vi "Demo_Main0.vi"() -> ()   [LabVIEW 2010]
uses:
  ControlCAN/ControlCAN.llb/DevType.ctl
  ControlCAN/ControlCAN.llb/CAN Channel.ctl
  ControlCAN/ControlCAN.llb/InitFlag.ctl
  ControlCAN/ControlCAN.llb/Mode.ctl
  ControlCAN/ControlCAN.llb/Fliter.ctl
  ControlCAN/ControlCAN.llb/VCI_CAN_OBJ.ctl
  ControlCAN/ControlCAN.llb/VCI_INIT_CONFIG.ctl
  ControlCAN/ControlCAN.llb/Return Val.ctl
  ControlCAN/ControlCAN.lvlib
panel:
  out "sCnt":u32 caption="处理统计"
  out "模式_回":string(combo)="00"
  in  "模式_R":bool
  in  "设定电流_R":bool
  in  "设定位置_R":bool
  in  "设定速度_R":bool
  in  "存储路径":path
  in  "保存":bool
  out "保存_S":bool
  in  "模式_W":bool
  in  "模式":string(combo)="00"
  in  "设定电流":dbl format="%#.6f"
  out "设定电流_回":dbl format="%#.6f"
  in  "设定电流_W":bool
  in  "设定位置":dbl format="%#.6f"
  out "设定位置_回":dbl format="%#.6f"
  in  "设定位置_W":bool
  in  "设定速度":dbl format="%#.1f"
  out "设定速度_回":dbl format="%#.6f"
  in  "设定速度_W":bool
  in  "监测_W":bool
  in  "监测":string(combo)="30"
  out "电机ID_R":u32
  in  "Clear":bool
  out "Ualfa":dbl format="%#.6f"
  out "Ubate":dbl format="%#.6f"
  out "Uq":dbl format="%#.6f"
  out "Ud":dbl format="%#.6f"
  out "PWM1":u16
  out "PWM2":u16
  out "PWM3":u16
  out "sector":u8
  out "Iqnow":dbl
  out "Idnow":dbl
  out "Ialfa":dbl
  out "Ibeta":dbl
  out "A电流":dbl
  out "C电流":dbl
  out "B电流":dbl
  out "供电电压":dbl
  out "机械角度":dbl format="%.2f"
  out "电气角度":dbl
  out "转速":dbl
  out "CAN STD_ID":u32 format="%x"
  in  "电机ID":string(combo)="00"
  in  "电机ID_W":bool
  out "RecvCnt":u32 caption="接收统计"
  out "SendCnt":u32 caption="发送统计"
  in  "Format":u8(ring) items=["标准帧", "扩展帧"]
  in  "Type":u8(ring) items=["数据帧", "远程帧"]
  in  "Data":string="00 01 02 03 04 05 06 07"
  in  "ID":u32=291 format="0x%x"
  in  "Send":bool
  in  "RcvEnable":bool=TRUE
  out "Open":bool
  in  "Fliter":T1=1 items=["接收所有类型"=1, "只接收标准帧"=2, "只接收扩展帧"=3]
  in  "kBaudRate":u8(ring)=12 caption="波特率" items=["5k bps"=1, "10k bps"=2, "20k bps"=3, "40k bps"=4, "50k bps"=5, "80k bps"=6, "100k bps"=7, "125k bps"=8, "200k bps"=9, "250k bps"=10, "400k bps"=11, "500k bps"=12, "666k bps"=13, "800k bps"=14, "1000k bps"=15, "33.33k bps"=16, "66.66k bps"=17, "83.33k bps"=18]
  in  "Mode":T2 caption="工作模式" items=["正常工作", "仅侦听模式", "自测模式（环回）"]
  in  "InitFlag":T3 caption="初始化参数" items=["使用Flash参数", "使用界面设置参数"]
  in  "AccMask":u32=4294967295 caption="接收屏蔽码" format="%08x"
  in  "AccCode":u32 caption="接收过滤码" format="%08x"
  in  "Close":bool
  in  "Open":bool
  in  "Channel":T4 caption="CAN通道" items=["通道1", "通道2"]
  in  "DevType":T5=3 caption="设备类型" items=["USB-CAN"=2, "USB-CAN2"=3]
  # "."
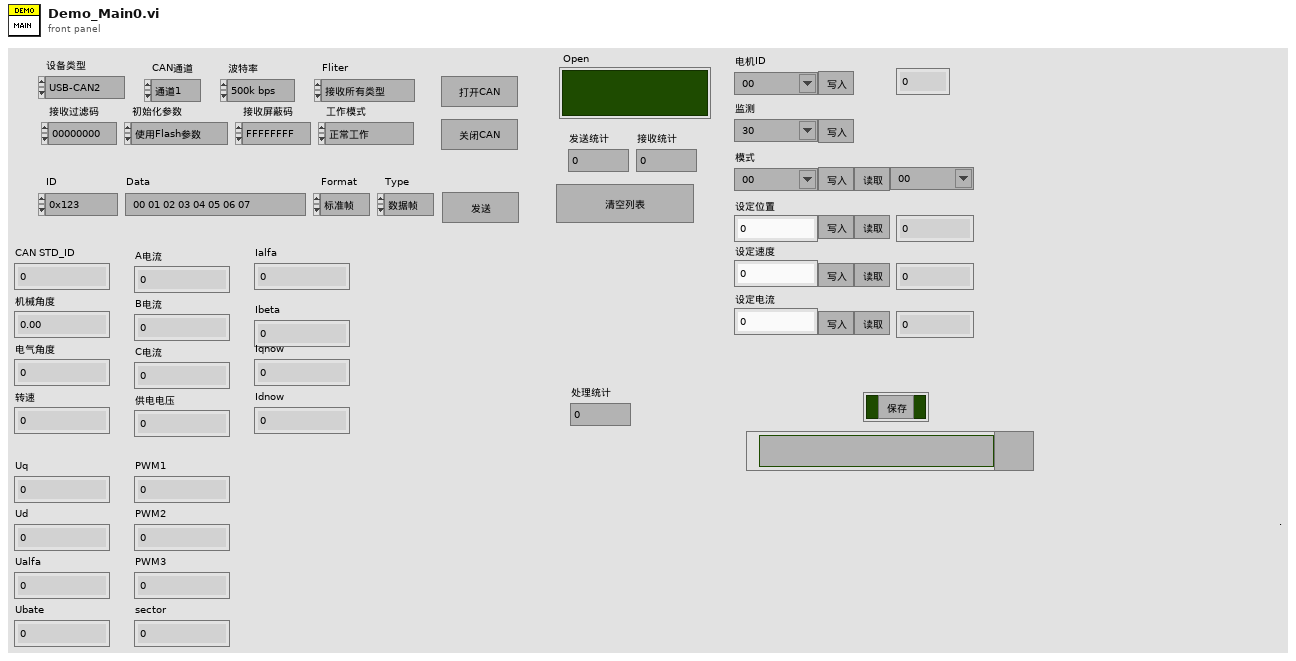
[diagram p1: front panel]
types:
  T1 = typedef "ControlCAN.lvlib/Fliter.ctl" = u8
  T2 = typedef "ControlCAN.lvlib/Mode.ctl" = u8
  T3 = typedef "ControlCAN.lvlib/InitFlag.ctl" = u32
  T4 = typedef "ControlCAN.lvlib/CAN Channel.ctl" = u32
  T5 = typedef "ControlCAN.lvlib/DevType.ctl" = u32
  T6 = typedef "ControlCAN.lvlib/VCI_CAN_OBJ.ctl" = cluster{"ID":u32, "TimeStamp":u32, "TimeFlag":u8, "SendType":u8, "RemoteFlag":u8, "ExternFlag":u8, "DataLen":u8, "Data":u8[], "Reserved":u8[]}
  T7 = cluster{"Type":enum16{"接收", "发送"}, "Channel":T4, "Time":timestamp, "VCI_CAN_OBJ":T6}[]
  T8 = typedef "ControlCAN.lvlib/VCI_INIT_CONFIG.ctl" = cluster{"AccCode":u32, "AccMask":u32, "InitFlag":T3, "Fliter":T1, "Timing0":u8, "Timing1":u8, "Mode":T2}
  T9 = cluster{"DevType":T5, "DevIndex":u32, "CanIndex":T4, "VCI_INIT_CONFIG":T8}
  T10 = typedef "ControlCAN.lvlib/Return Val.ctl" = i32
  T11 = enum16{"open", "replace", "create", "open or create", "replace or create", "replace or create with confirmation"}
  T12 = cluster{"[0]":cluster{"Type":enum16{"接收", "发送"}, "Channel":T4, "Time":timestamp, "VCI_CAN_OBJ":T6}}
  T13 = cluster{"Type":enum16{"接收", "发送"}, "Channel":T4, "Time":timestamp, "VCI_CAN_OBJ":T6}
  T14 = cluster{"Data[0]":u8, "Data[1]":u8, "Data[2]":u8, "Data[3]":u8, "Data[4]":u8, "Data[5]":u8, "Data[6]":u8, "Data[7]":u8}
  T15 = enum32{"invalid app kind", "Development System", "Run Time System", "Student Edition", "Embedded LabVIEW", "Evaluation", "Custom"}
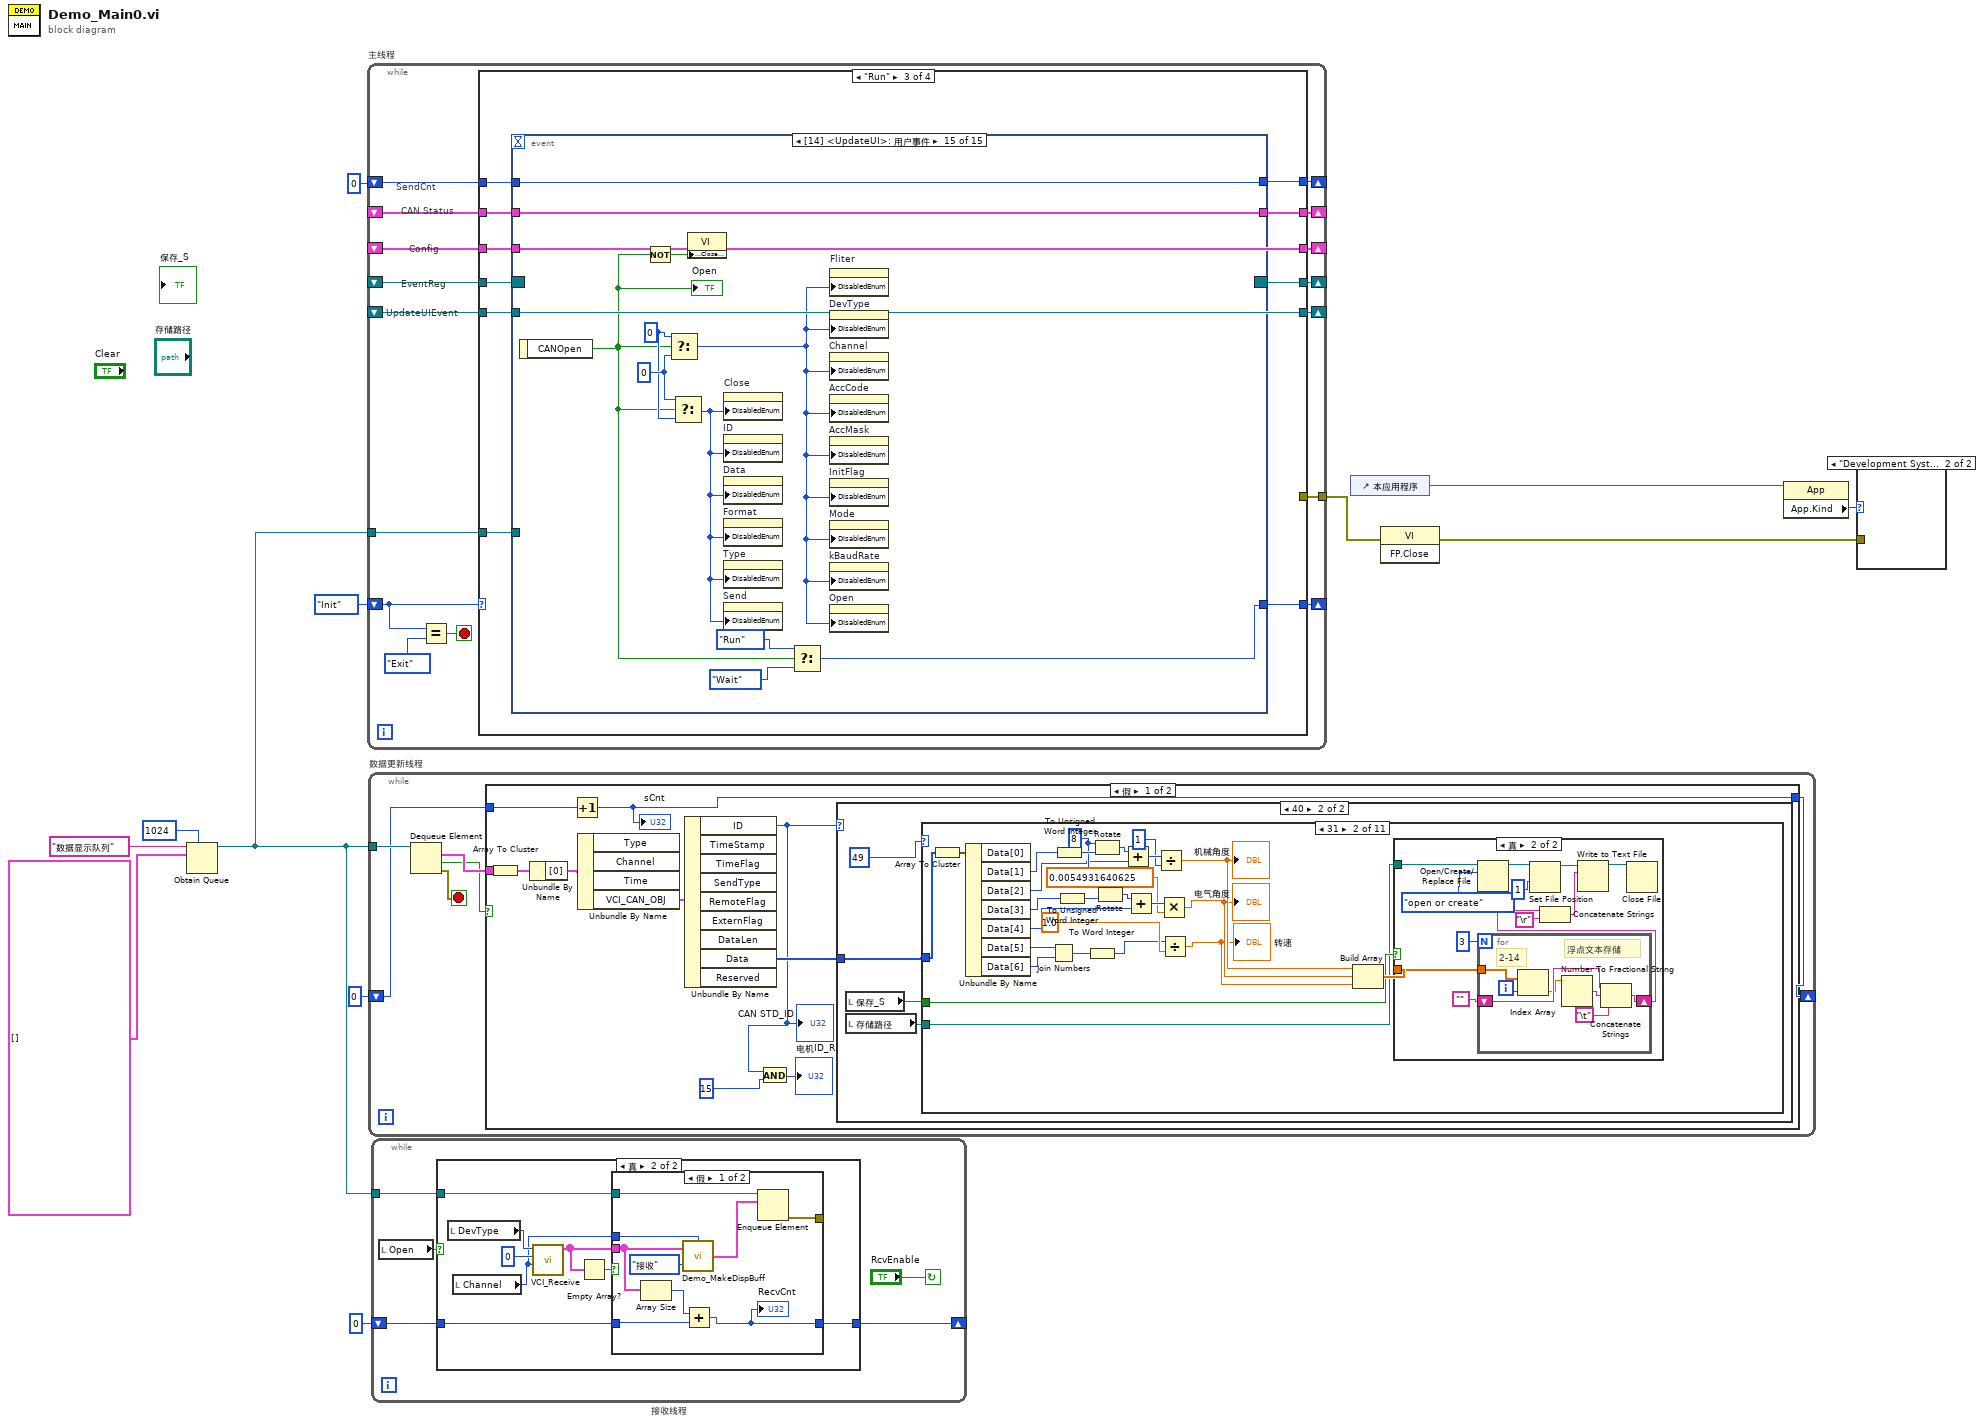
[diagram p0: block diagram]
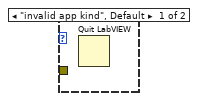
[diagram p2: hidden frame]
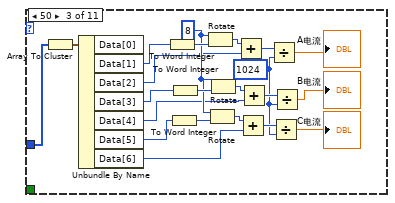
[diagram p6: hidden frame]
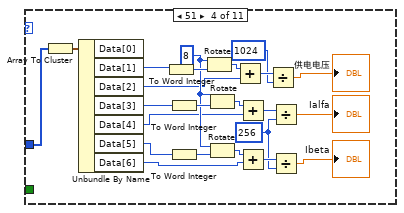
[diagram p7: hidden frame]
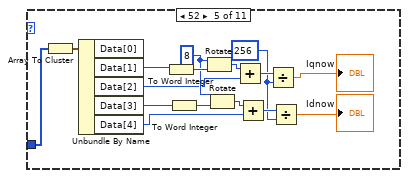
[diagram p8: hidden frame]
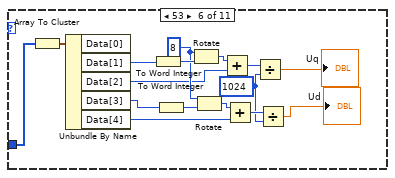
[diagram p9: hidden frame]
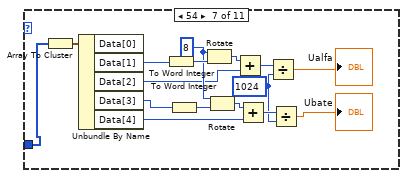
[diagram p10: hidden frame]
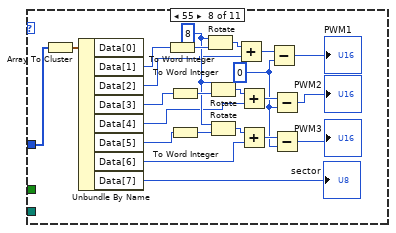
[diagram p11: hidden frame]
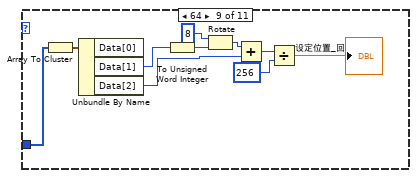
[diagram p12: hidden frame]
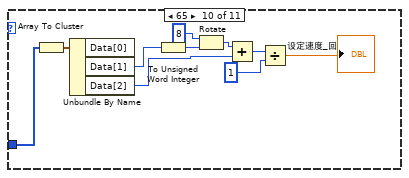
[diagram p13: hidden frame]
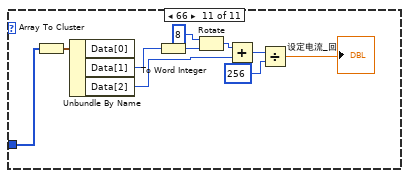
[diagram p14: hidden frame]
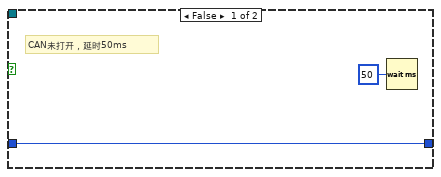
[diagram p16: hidden frame]
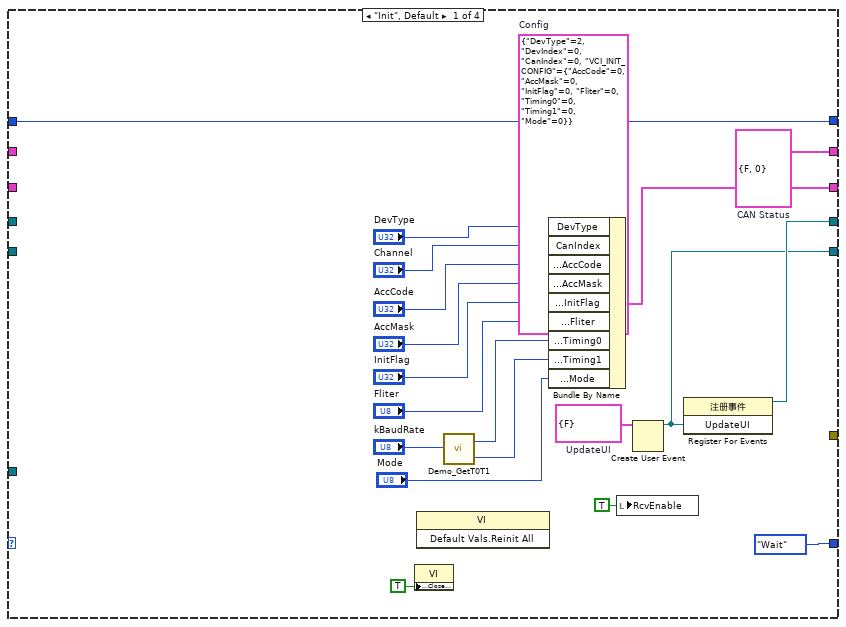
[diagram p18: hidden frame]
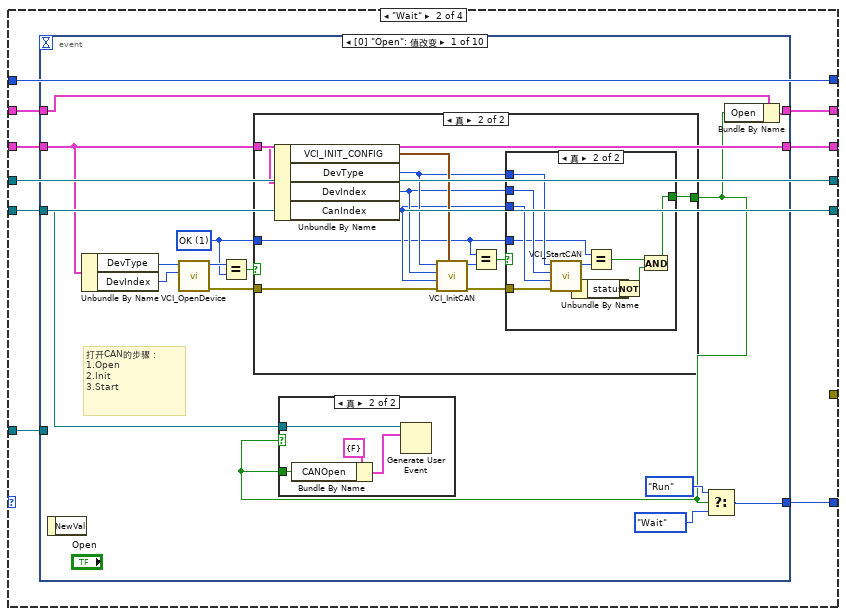
[diagram p19: hidden frame]
diagram:
  n1 = Obtain Queue(max queue size (-1, unlimited)=1024, name (unnamed)="数据显示队列" ("名称（未命名）"), element data type=T7 []) -> (queue out=w9:refnum<queue>)  [unwired: 2 in, 2 out]
  n2 = while "主线程" {
    shift-right: [w24] -> _
    shift-left: enum16{"Init", "Wait", "Run", "Exit"}."Init" -> [w27]
    shift-right: [w25] -> _
    shift-left: _ -> [w26]
    shift-right: [w23] -> _
    shift-left: _ -> [w22]
    tunnel: w9 -> [w21]
    shift-right: [w19] -> _
    shift-left: _ -> [w18]
    shift-right: [w17] -> _
    shift-left: _ -> [w16]
    shift-right: [w14] -> _
    shift-left: u32 0 -> [w15]
    tunnel: [w13] -> w4
    stop <- w28 stop-if-true
    # "CAN Status"
    # "Config"
    # "EventReg"
    # "UpdateUIEvent"
    # "SendCnt"
    n3 = Equal?(x=w27, y=enum16{"Init", "Wait", "Run", "Exit"}."Exit") -> (x = y?=w28:bool)
    n4 = case shown="\"Run\"" w27 {
      tunnel: w26 -> [_ w57 w156 w459]
      tunnel: [w48 w56 w155 w459] -> w25
      tunnel: [enum16{"Init", "Wait", "Run", "Exit"}."Wait" w53 w158 enum16{"Init", "Wait", "Run", "Exit"}."Exit"] -> w24
      tunnel: [w44 w54 w154 w457] -> w23
      tunnel: w22 -> [_ w55 w154 w457]
      tunnel: w21 -> [_ w52 w157 w463]
      tunnel: [w36 w51 w152 w462] -> w19
      tunnel: w18 -> [_ w51 w153 w462]
      tunnel: [w35 w50 w151 w460] -> w17
      tunnel: w16 -> [_ w50 w151 w460]
      tunnel: w15 -> [w33 w49 w150 w455]
      tunnel: [w33 w49 w149 w455] -> w14
      tunnel: [_ _ _ errorcluster {"status"=FALSE, "code"=0, "source"=""} ("error constant")] -> w13
      frame "Init", Default {
        w37 = cluster{"CANOpen":bool} {"CANOpen"=FALSE}  # UpdateUI
        w47 = T9 {"DevType"=2, "DevIndex"=0, "CanIndex"=0, "VCI_INIT_CONFIG"={"AccCode"=0, "AccMask"=0, "InitFlag"=0, "Fliter"=0, "Timing0"=0, "Timing1"=0, "Mode"=0}}  # Config
        w48 = cluster{"Open":bool, "SendCnt":u32} {"Open"=FALSE, "SendCnt"=0}  # CAN Status
        n5 = property class="VI"("Front Panel.Closeable"=TRUE ("前面板窗口:可关闭")) -> ()  [unwired: 2 in, 2 out]
        n6 = invoke class="VI" method="Default Vals.Reinit All"() -> ()  [unwired: 3 in, 3 out]
        n7 = call "Demo_GetT0T1.vi"("kBaudRate"="kBaudRate") -> ("Timing0"=w30:u8, "Timing1"=w29:u8)
        n8 = Bundle By Name(cluster=w47, "DevType"="DevType", "CanIndex"="Channel", "VCI_INIT_CONFIG.AccCode"="AccCode", "VCI_INIT_CONFIG.AccMask"="AccMask", "VCI_INIT_CONFIG.InitFlag"="InitFlag", "VCI_INIT_CONFIG.Fliter"="Fliter", "VCI_INIT_CONFIG.Timing0"=w30, "VCI_INIT_CONFIG.Timing1"=w29, "VCI_INIT_CONFIG.Mode"="Mode") -> (w44:T9)
        n9 = local write "RcvEnable"(TRUE ("RcvEnable")) -> ()
        n10 = Create User Event(user event datatype=w37) -> (user event=w35:refnum<user-event>)  [unwired: 1 in, 1 out]
        n11 = register-events(w35) -> (reference out=w36:refnum<event-registration>)  [unwired: 2 in, 1 out]
      }
      frame "Wait" {
        n12 = event shown="[0] \"Open\": 值改变" {
          selector: _ -> [_ _ _ _ _ _ _ _ _ _]
          dyn-events: _ -> [_ _ _ _ _ _ _ _ _ _]
          timeout: _ -> [_ _ _ _ _ _ _ _ _ _]
          tunnel: w57 -> [w61 w101 w111 w116 w121 w126 w131 w136 w143 w148]
          tunnel: [w60 w101 w111 w116 w121 w126 w131 w136 w143 w148] -> w56
          tunnel: w55 -> [w71 w100 w110 w115 w120 w125 w130 w135 w142 w147]
          tunnel: [w71 w100 w109 w113 w118 w123 w128 w133 w141 w145] -> w54
          tunnel: [w62 enum16{"Init", "Wait", "Run", "Exit"}."Exit" enum16{"Init", "Wait", "Run", "Exit"}."Wait" enum16{"Init", "Wait", "Run", "Exit"}."Wait" enum16{"Init", "Wait", "Run", "Exit"}."Wait" enum16{"Init", "Wait", "Run", "Exit"}."Wait" enum16{"Init", "Wait", "Run", "Exit"}."Wait" enum16{"Init", "Wait", "Run", "Exit"}."Wait" enum16{"Init", "Wait", "Run", "Exit"}."Wait" enum16{"Init", "Wait", "Run", "Exit"}."Wait"] -> w53
          tunnel: w52 -> [_ _ _ _ _ _ _ _ _ _]
          tunnel: w50 -> [w59 _ _ _ _ _ _ _ _ _]
          event "Open": Value Change {
            w65 = T10 1 items=["OK"=1, "ERROR1"=0, "ERROR2"=-1] ("y")
            # "打开CAN的步骤：\n1.Open\n2.Init\n3.Start"
            n13 = event-data() -> ()  [unwired: 2 out]
            n14 = Unbundle By Name(w71) -> ("DevType"=w70:T5, "DevIndex"=w69:u32)
            n15 = call "VCI_OpenDevice.vi"("DevIndex"=w69, "DevType"=w70) -> ("error out"=w66:errorcluster, "Return Val"=w68:T10)  [unwired: 2 in, 6 out]
            n16 = Equal?(x=w68, y=w65) -> (x = y?=w67:bool)
            n17 = case shown="真" w67 {
              tunnel: w66 -> [_ w86]
              tunnel: w71 -> [_ w85]
              tunnel: w65 -> [_ w77]
              tunnel: [_ w76] -> w58
              frame False {
              }
              frame True {
                n18 = Unbundle By Name(w85) -> ("VCI_INIT_CONFIG"=w84:T8, "DevType"=w80:T5, "DevIndex"=w79:u32, "CanIndex"=w78:T4)
                n19 = call "VCI_InitCAN.vi"("VCI_INIT_CONFIG"=w84, "error in (no error)"=w86, "CANIndex"=w78, "DevIndex"=w79, "DevType"=w80) -> ("error out"=w81:errorcluster, "Return Val"=w83:T10)  [unwired: 5 out]
                n20 = Equal?(x=w77, y=w83) -> (x = y?=w82:bool)
                n21 = case shown="真" w82 {
                  tunnel: w81 -> [_ w97]
                  tunnel: w80 -> [_ w96]
                  tunnel: w79 -> [_ w95]
                  tunnel: w78 -> [_ w94]
                  tunnel: w77 -> [_ w92]
                  tunnel: [_ w88] -> w76
                  frame False {
                  }
                  frame True {
                    n22 = call "VCI_StartCAN.vi"("error in (no error)"=w97, "CANIndex"=w94, "DevIndex"=w95, "DevType"=w96) -> ("error out"=w90:errorcluster, "Return Val"=w93:T10)  [unwired: 6 out]
                    n23 = Unbundle By Name(w90) -> ("status"=w87:bool)
                    n24 = Equal?(x=w92, y=w93) -> (x = y?=w91:bool)
                    n25 = Not(x=w87) -> (.not. x?=w89:bool)
                    n26 = And(x=w91, y=w89) -> (x .and. y?=w88:bool)
                  }
                }
              }
            }
            n27 = case shown="真" w58 {
              tunnel: w59 -> [_ w75]
              tunnel: w58 -> [_ w73]
              frame False {
              }
              frame True {
                n28 = Bundle By Name(cluster=cluster{"CANOpen":bool} {"CANOpen"=FALSE} ("事件数据"), "CANOpen"=w73) -> (w72:cluster{"CANOpen":bool})
                n29 = Generate User Event(user event=w75, event data cluster=w72) -> ()  [unwired: 1 in, 2 out]
              }
            }
            n30 = Select(t=enum16{"Init", "Wait", "Run", "Exit"}."Run", s=w58, f=enum16{"Init", "Wait", "Run", "Exit"}."Wait") -> (s? t:f=w62:enum16{"Init", "Wait", "Run", "Exit"})
            n31 = Bundle By Name(cluster=w61, "Open"=w58) -> (w60:cluster{"Open":bool, "SendCnt":u32})
          }
          event Panel Close? {
            n32 = event-data() -> ()  [unwired: 2 out]
            n33 = event-data("Discard?"=TRUE ("放弃？")) -> ()  [unwired: 1 in, 1 out]
          }
          event Value Change {
            w107 = T5 3 items=["USB-CAN"=2, "USB-CAN2"=3] ("y")
            n34 = event-data() -> ("NewVal"=w108:T5)  [unwired: 1 out]
            n35 = Equal?(x=w108, y=w107) -> (x = y?=w106:bool)
            n36 = Bundle By Name(cluster=w110, "DevType"=w108) -> (w109:T9)
            n37 = Select(t=i32[] [] ("禁用项[]"), s=w106, f=i32[] [1] ("禁用项[]")) -> (s? t:f=w105:i32[])
            n38 = property on="Channel" class="Ring (严格)"("Disabled Items []"=w105) -> ()  [unwired: 2 in, 2 out]
          }
          event Value Change {
            n39 = event-data() -> ("NewVal"=w114:T4)  [unwired: 1 out]
            n40 = Bundle By Name(cluster=w115, "CanIndex"=w114) -> (w113:T9)
          }
          event "AccCode": Value Change {
            n41 = event-data() -> ("NewVal"=w119:u32)  [unwired: 1 out]
            n42 = Bundle By Name(cluster=w120, "VCI_INIT_CONFIG.AccCode"=w119) -> (w118:T9)
          }
          event "AccMask": Value Change {
            n43 = event-data() -> ("NewVal"=w124:u32)  [unwired: 1 out]
            n44 = Bundle By Name(cluster=w125, "VCI_INIT_CONFIG.AccMask"=w124) -> (w123:T9)
          }
          event Value Change {
            n45 = event-data() -> ("NewVal"=w129:T3)  [unwired: 1 out]
            n46 = Bundle By Name(cluster=w130, "VCI_INIT_CONFIG.InitFlag"=w129) -> (w128:T9)
          }
          event Value Change {
            n47 = event-data() -> ("NewVal"=w134:T2)  [unwired: 1 out]
            n48 = Bundle By Name(cluster=w135, "VCI_INIT_CONFIG.Mode"=w134) -> (w133:T9)
          }
          event "kBaudRate": Value Change {
            n49 = event-data() -> ("NewVal"=w139:u8)  [unwired: 1 out]
            n50 = call "Demo_GetT0T1.vi"("kBaudRate"=w139) -> ("Timing0"=w138:u8, "Timing1"=w137:u8)
            n51 = Bundle By Name(cluster=w142, "VCI_INIT_CONFIG.Timing0"=w138, "VCI_INIT_CONFIG.Timing1"=w137) -> (w141:T9)
          }
          event Value Change {
            n52 = event-data() -> ("NewVal"=w146:T1)  [unwired: 1 out]
            n53 = Bundle By Name(cluster=w147, "VCI_INIT_CONFIG.Fliter"=w146) -> (w145:T9)
          }
        }
      }
      frame "Run" {
        n54 = event shown="[14] <UpdateUI>: 用户事件" {
          selector: w153 -> [_ _ _ _ _ _ _ _ _ _ _ _ _ _ _]
          dyn-events: [_ _ _ _ _ _ _ _ _ _ _ _ _ _ _] -> w152
          timeout: _ -> [_ _ _ _ _ _ _ _ _ _ _ _ _ _ _]
          tunnel: [enum16{"Init", "Wait", "Run", "Exit"}."Run" enum16{"Init", "Wait", "Run", "Exit"}."Run" enum16{"Init", "Wait", "Run", "Exit"}."Run" enum16{"Init", "Wait", "Run", "Exit"}."Run" enum16{"Init", "Wait", "Run", "Exit"}."Run" enum16{"Init", "Wait", "Run", "Exit"}."Run" enum16{"Init", "Wait", "Run", "Exit"}."Run" enum16{"Init", "Wait", "Run", "Exit"}."Run" enum16{"Init", "Wait", "Run", "Exit"}."Run" enum16{"Init", "Wait", "Run", "Exit"}."Run" enum16{"Init", "Wait", "Run", "Exit"}."Run" enum16{"Init", "Wait", "Run", "Exit"}."Run" enum16{"Init", "Wait", "Run", "Exit"}."Run" enum16{"Init", "Wait", "Run", "Exit"}."Run" w447] -> w158
          tunnel: w157 -> [_ _ _ _ _ _ _ _ _ _ _ _ _ _ _]
          tunnel: [w160 w177 w194 w215 w238 w259 w285 w311 w337 w358 w379 w400 w428 w434 w453] -> w155
          tunnel: w156 -> [w160 w177 w194 w215 w238 w259 w285 w311 w337 w358 w379 w400 w428 w436 w453]
          tunnel: w154 -> [_ w172 w183 w204 w218 w240 w269 w291 w317 w339 w360 w381 _ w441 _]
          tunnel: w151 -> [_ _ _ _ _ _ _ _ _ _ _ _ _ w433 _]
          tunnel: w150 -> [w159 w165 w193 w214 w237 w258 w284 w310 w336 w357 w378 w399 w427 w429 w446]
          tunnel: [w159 w164 w193 w214 w237 w258 w284 w310 w336 w357 w378 w399 w427 w429 w446] -> w149
          event Timeout {
            n55 = event-data() -> ()  [unwired: 3 out]
          }
          event "Send": Value Change {
            n56 = event-data() -> ()  [unwired: 2 out]
            n57 = Increment(x=w165) -> (x+1=w164:u32)
            "SendCnt" <- w164
            n58 = call "Demo_MakeData.vi"("DataString"="Data") -> ("Data"=w167:u8[], "DataLen"=w168:u8)  [unwired: 9 out]
            n59 = Bundle By Name(cluster=T6 {"ID"=0, "TimeStamp"=0, "TimeFlag"=0, "SendType"=0, "RemoteFlag"=0, "ExternFlag"=0, "DataLen"=0, "Data"=[], "Reserved"=[]} ("Send"), "ID"="ID", "RemoteFlag"="Type", "ExternFlag"="Format", "DataLen"=w168, "Data"=w167) -> (w162:T6)
            n60 = Build Array(w162) -> (w163:T6[])
            n61 = Unbundle By Name(w172) -> ("DevType"=w171:T5, "DevIndex"=w170:u32, "CanIndex"=w166:T4)
            n62 = call "VCI_Transmit.vi"("Buffer"=w163, "CANIndex"=w166, "DevIndex"=w170, "DevType"=w171) -> ()  [unwired: 1 in, 7 out]
          }
          event "电机ID_W": Value Change {
            w181 = u8 0 items=["数据帧", "遥控帧"]
            w180 = u8 0 items=["标准帧", "扩展帧"]
            n63 = event-data() -> ()  [unwired: 2 out]
            n64 = call "Demo_MakeData.vi"("DataString"="电机ID") -> ("Data"=w187:u8[], "DataLen"=w188:u8)  [unwired: 9 out]
            n65 = Bundle By Name(cluster=T6 {"ID"=0, "TimeStamp"=0, "TimeFlag"=0, "SendType"=0, "RemoteFlag"=0, "ExternFlag"=0, "DataLen"=0, "Data"=[], "Reserved"=[]} ("Send"), "ID"=u32 138, "RemoteFlag"=w181, "ExternFlag"=w180, "DataLen"=w188, "Data"=w187) -> (w184:T6)
            n66 = Build Array(w184) -> (w185:T6[])
            n67 = Unbundle By Name(w183) -> ("DevType"=w190:T5, "DevIndex"=w189:u32, "CanIndex"=w186:T4)
            n68 = call "VCI_Transmit.vi"("Buffer"=w185, "CANIndex"=w186, "DevIndex"=w189, "DevType"=w190) -> ()  [unwired: 1 in, 7 out]
          }
          event "监测_W": Value Change {
            w212 = u8 0 items=["数据帧", "遥控帧"]
            w213 = u8 0 items=["标准帧", "扩展帧"]
            # "地址"
            n69 = event-data() -> ()  [unwired: 2 out]
            n70 = property on="电机ID" class="CmbBox"() -> ("Value"=w201:string)  [unwired: 2 in, 2 out]
            n71 = Scan From String(format string="%x" ("格式字符串"), input string=w201, default 1=u8 0) -> (output 1=w197:u8)  [unwired: 2 in, 3 out]
            n72 = call "Demo_MakeData.vi"("DataString"="监测") -> ("Data"=w196:u8[], "DataLen"=w208:u8)  [unwired: 9 out]
            n73 = Add(x=u32 48, y=w197) -> (x+y=w199:u32)
            n74 = Bundle By Name(cluster=T6 {"ID"=0, "TimeStamp"=0, "TimeFlag"=0, "SendType"=0, "RemoteFlag"=0, "ExternFlag"=0, "DataLen"=0, "Data"=[], "Reserved"=[]} ("Send"), "ID"=w199, "RemoteFlag"=w212, "ExternFlag"=w213, "DataLen"=w208, "Data"=w196) -> (w211:T6)
            n75 = Build Array(w211) -> (w210:T6[])
            n76 = Unbundle By Name(w204) -> ("DevType"=w206:T5, "DevIndex"=w207:u32, "CanIndex"=w209:T4)
            n77 = call "VCI_Transmit.vi"("Buffer"=w210, "CANIndex"=w209, "DevIndex"=w207, "DevType"=w206) -> ()  [unwired: 1 in, 7 out]
          }
          event "模式_W": Value Change {
            w220 = u8 0 items=["数据帧", "遥控帧"]
            w219 = u8 0 items=["标准帧", "扩展帧"]
            # "地址"
            n78 = event-data() -> ()  [unwired: 2 out]
            n79 = property on="电机ID" class="CmbBox"() -> ("Value"=w229:string)  [unwired: 2 in, 2 out]
            n80 = Concatenate Strings("20 ", "模式") -> (w234:string)
            n81 = Scan From String(format string="%x" ("格式字符串"), input string=w229, default 1=u8 0) -> (output 1=w233:u8)  [unwired: 2 in, 3 out]
            n82 = call "Demo_MakeData.vi"("DataString"=w234) -> ("Data"=w236:u8[], "DataLen"=w224:u8)  [unwired: 9 out]
            n83 = Add(x=u32 16, y=w233) -> (x+y=w231:u32)
            n84 = Bundle By Name(cluster=T6 {"ID"=0, "TimeStamp"=0, "TimeFlag"=0, "SendType"=0, "RemoteFlag"=0, "ExternFlag"=0, "DataLen"=0, "Data"=[], "Reserved"=[]} ("Send"), "ID"=w231, "RemoteFlag"=w220, "ExternFlag"=w219, "DataLen"=w224, "Data"=w236) -> (w221:T6)
            n85 = Build Array(w221) -> (w222:T6[])
            n86 = Unbundle By Name(w218) -> ("DevType"=w226:T5, "DevIndex"=w225:u32, "CanIndex"=w223:T4)
            n87 = call "VCI_Transmit.vi"("Buffer"=w222, "CANIndex"=w223, "DevIndex"=w225, "DevType"=w226) -> ()  [unwired: 1 in, 7 out]
            "模式_回" <- "模式"
          }
          event "模式_R": Value Change {
            w255 = u8 0 items=["数据帧", "遥控帧"]
            w256 = u8 0 items=["标准帧", "扩展帧"]
            # "地址"
            n88 = event-data() -> ()  [unwired: 2 out]
            n89 = property on="电机ID" class="CmbBox"() -> ("Value"=w246:string)  [unwired: 2 in, 2 out]
            n90 = Scan From String(format string="%x" ("格式字符串"), input string=w246, default 1=u8 0) -> (output 1=w242:u8)  [unwired: 2 in, 3 out]
            n91 = call "Demo_MakeData.vi"("DataString"="20 ") -> ("Data"=w241:u8[], "DataLen"=w251:u8)  [unwired: 9 out]
            n92 = Add(x=u32 48, y=w242) -> (x+y=w244:u32)
            n93 = Bundle By Name(cluster=T6 {"ID"=0, "TimeStamp"=0, "TimeFlag"=0, "SendType"=0, "RemoteFlag"=0, "ExternFlag"=0, "DataLen"=0, "Data"=[], "Reserved"=[]} ("Send"), "ID"=w244, "RemoteFlag"=w255, "ExternFlag"=w256, "DataLen"=w251, "Data"=w241) -> (w254:T6)
            n94 = Build Array(w254) -> (w253:T6[])
            n95 = Unbundle By Name(w240) -> ("DevType"=w249:T5, "DevIndex"=w250:u32, "CanIndex"=w252:T4)
            n96 = call "VCI_Transmit.vi"("Buffer"=w253, "CANIndex"=w252, "DevIndex"=w250, "DevType"=w249) -> ()  [unwired: 1 in, 7 out]
          }
          event "设定位置_W": Value Change {
            w271 = u8 0 items=["数据帧", "遥控帧"]
            w270 = u8 0 items=["标准帧", "扩展帧"]
            # "索引地址"
            n97 = event-data() -> ()  [unwired: 2 out]
            n98 = property on="电机ID" class="CmbBox"() -> ("Value"=w279:string)  [unwired: 2 in, 2 out]
            n99 = Multiply ("乘")(x="设定位置", y=u16 256) -> (x*y=w262:i16)
            n100 = Scan From String(format string="%x" ("格式字符串"), input string=w279, default 1=u8 0) -> (output 1=w283:u8)  [unwired: 2 in, 3 out]
            n101 = Split Number(x=w262) -> (hi(x)=w261:u8, lo(x)=w260:u8)
            n102 = Add(x=u32 16, y=w283) -> (x+y=w281:u32)
            n103 = Build Array(u8 64, w261, w260) -> (w265:u8[])
            n104 = Bundle By Name(cluster=T6 {"ID"=0, "TimeStamp"=0, "TimeFlag"=0, "SendType"=0, "RemoteFlag"=0, "ExternFlag"=0, "DataLen"=0, "Data"=[], "Reserved"=[]} ("Send"), "ID"=w281, "RemoteFlag"=w271, "ExternFlag"=w270, "DataLen"=u8 3, "Data"=w265) -> (w272:T6)
            n105 = Build Array(w272) -> (w273:T6[])
            n106 = Unbundle By Name(w269) -> ("DevType"=w276:T5, "DevIndex"=w275:u32, "CanIndex"=w274:T4)
            n107 = call "VCI_Transmit.vi"("Buffer"=w273, "CANIndex"=w274, "DevIndex"=w275, "DevType"=w276) -> ()  [unwired: 1 in, 7 out]
          }
          event "设定速度_W": Value Change {
            w304 = u8 0 items=["数据帧", "遥控帧"]
            w305 = u8 0 items=["标准帧", "扩展帧"]
            # "索引地址"
            n108 = event-data() -> ()  [unwired: 2 out]
            n109 = property on="电机ID" class="CmbBox"() -> ("Value"=w296:string)  [unwired: 2 in, 2 out]
            n110 = Multiply ("乘")(x="设定速度", y=i16 1) -> (x*y=w288:i16)
            n111 = Scan From String(format string="%x" ("格式字符串"), input string=w296, default 1=u8 0) -> (output 1=w292:u8)  [unwired: 2 in, 3 out]
            n112 = Split Number(x=w288) -> (hi(x)=w287:u8, lo(x)=w286:u8)
            n113 = Add(x=u32 16, y=w292) -> (x+y=w294:u32)
            n114 = Build Array(u8 65, w287, w286) -> (w308:u8[])
            n115 = Bundle By Name(cluster=T6 {"ID"=0, "TimeStamp"=0, "TimeFlag"=0, "SendType"=0, "RemoteFlag"=0, "ExternFlag"=0, "DataLen"=0, "Data"=[], "Reserved"=[]} ("Send"), "ID"=w294, "RemoteFlag"=w304, "ExternFlag"=w305, "DataLen"=u8 3, "Data"=w308) -> (w303:T6)
            n116 = Build Array(w303) -> (w302:T6[])
            n117 = Unbundle By Name(w291) -> ("DevType"=w299:T5, "DevIndex"=w300:u32, "CanIndex"=w301:T4)
            n118 = call "VCI_Transmit.vi"("Buffer"=w302, "CANIndex"=w301, "DevIndex"=w300, "DevType"=w299) -> ()  [unwired: 1 in, 7 out]
          }
          event "设定电流_W": Value Change {
            w323 = u8 0 items=["数据帧", "遥控帧"]
            w322 = u8 0 items=["标准帧", "扩展帧"]
            # "索引地址"
            n119 = event-data() -> ()  [unwired: 2 out]
            n120 = property on="电机ID" class="CmbBox"() -> ("Value"=w331:string)  [unwired: 2 in, 2 out]
            n121 = Multiply ("乘")(x="设定电流", y=i16 256) -> (x*y=w314:i16)
            n122 = Scan From String(format string="%x" ("格式字符串"), input string=w331, default 1=u8 0) -> (output 1=w335:u8)  [unwired: 2 in, 3 out]
            n123 = Split Number(x=w314) -> (hi(x)=w313:u8, lo(x)=w312:u8)
            n124 = Add(x=u32 16, y=w335) -> (x+y=w333:u32)
            n125 = Build Array(u8 66, w313, w312) -> (w319:u8[])
            n126 = Bundle By Name(cluster=T6 {"ID"=0, "TimeStamp"=0, "TimeFlag"=0, "SendType"=0, "RemoteFlag"=0, "ExternFlag"=0, "DataLen"=0, "Data"=[], "Reserved"=[]} ("Send"), "ID"=w333, "RemoteFlag"=w323, "ExternFlag"=w322, "DataLen"=u8 3, "Data"=w319) -> (w324:T6)
            n127 = Build Array(w324) -> (w325:T6[])
            n128 = Unbundle By Name(w317) -> ("DevType"=w328:T5, "DevIndex"=w327:u32, "CanIndex"=w326:T4)
            n129 = call "VCI_Transmit.vi"("Buffer"=w325, "CANIndex"=w326, "DevIndex"=w327, "DevType"=w328) -> ()  [unwired: 1 in, 7 out]
          }
          event "设定位置_R": Value Change {
            w342 = u8 0 items=["数据帧", "遥控帧"]
            w341 = u8 0 items=["标准帧", "扩展帧"]
            # "地址"
            n130 = event-data() -> ()  [unwired: 2 out]
            n131 = property on="电机ID" class="CmbBox"() -> ("Value"=w351:string)  [unwired: 2 in, 2 out]
            n132 = Scan From String(format string="%x" ("格式字符串"), input string=w351, default 1=u8 0) -> (output 1=w355:u8)  [unwired: 2 in, 3 out]
            n133 = call "Demo_MakeData.vi"("DataString"="40 ") -> ("Data"=w356:u8[], "DataLen"=w346:u8)  [unwired: 9 out]
            n134 = Add(x=u32 48, y=w355) -> (x+y=w353:u32)
            n135 = Bundle By Name(cluster=T6 {"ID"=0, "TimeStamp"=0, "TimeFlag"=0, "SendType"=0, "RemoteFlag"=0, "ExternFlag"=0, "DataLen"=0, "Data"=[], "Reserved"=[]} ("Send"), "ID"=w353, "RemoteFlag"=w342, "ExternFlag"=w341, "DataLen"=w346, "Data"=w356) -> (w343:T6)
            n136 = Build Array(w343) -> (w344:T6[])
            n137 = Unbundle By Name(w339) -> ("DevType"=w348:T5, "DevIndex"=w347:u32, "CanIndex"=w345:T4)
            n138 = call "VCI_Transmit.vi"("Buffer"=w344, "CANIndex"=w345, "DevIndex"=w347, "DevType"=w348) -> ()  [unwired: 1 in, 7 out]
          }
          event "设定速度_R": Value Change {
            w375 = u8 0 items=["数据帧", "遥控帧"]
            w376 = u8 0 items=["标准帧", "扩展帧"]
            # "地址"
            n139 = event-data() -> ()  [unwired: 2 out]
            n140 = property on="电机ID" class="CmbBox"() -> ("Value"=w366:string)  [unwired: 2 in, 2 out]
            n141 = Scan From String(format string="%x" ("格式字符串"), input string=w366, default 1=u8 0) -> (output 1=w362:u8)  [unwired: 2 in, 3 out]
            n142 = call "Demo_MakeData.vi"("DataString"="41 ") -> ("Data"=w361:u8[], "DataLen"=w371:u8)  [unwired: 9 out]
            n143 = Add(x=u32 48, y=w362) -> (x+y=w364:u32)
            n144 = Bundle By Name(cluster=T6 {"ID"=0, "TimeStamp"=0, "TimeFlag"=0, "SendType"=0, "RemoteFlag"=0, "ExternFlag"=0, "DataLen"=0, "Data"=[], "Reserved"=[]} ("Send"), "ID"=w364, "RemoteFlag"=w375, "ExternFlag"=w376, "DataLen"=w371, "Data"=w361) -> (w374:T6)
            n145 = Build Array(w374) -> (w373:T6[])
            n146 = Unbundle By Name(w360) -> ("DevType"=w369:T5, "DevIndex"=w370:u32, "CanIndex"=w372:T4)
            n147 = call "VCI_Transmit.vi"("Buffer"=w373, "CANIndex"=w372, "DevIndex"=w370, "DevType"=w369) -> ()  [unwired: 1 in, 7 out]
          }
          event "设定电流_R": Value Change {
            w396 = u8 0 items=["数据帧", "遥控帧"]
            w397 = u8 0 items=["标准帧", "扩展帧"]
            # "地址"
            n148 = event-data() -> ()  [unwired: 2 out]
            n149 = property on="电机ID" class="CmbBox"() -> ("Value"=w387:string)  [unwired: 2 in, 2 out]
            n150 = Scan From String(format string="%x" ("格式字符串"), input string=w387, default 1=u8 0) -> (output 1=w383:u8)  [unwired: 2 in, 3 out]
            n151 = call "Demo_MakeData.vi"("DataString"="42 ") -> ("Data"=w382:u8[], "DataLen"=w392:u8)  [unwired: 9 out]
            n152 = Add(x=u32 48, y=w383) -> (x+y=w385:u32)
            n153 = Bundle By Name(cluster=T6 {"ID"=0, "TimeStamp"=0, "TimeFlag"=0, "SendType"=0, "RemoteFlag"=0, "ExternFlag"=0, "DataLen"=0, "Data"=[], "Reserved"=[]} ("Send"), "ID"=w385, "RemoteFlag"=w396, "ExternFlag"=w397, "DataLen"=w392, "Data"=w382) -> (w395:T6)
            n154 = Build Array(w395) -> (w394:T6[])
            n155 = Unbundle By Name(w381) -> ("DevType"=w390:T5, "DevIndex"=w391:u32, "CanIndex"=w393:T4)
            n156 = call "VCI_Transmit.vi"("Buffer"=w394, "CANIndex"=w393, "DevIndex"=w391, "DevType"=w390) -> ()  [unwired: 1 in, 7 out]
          }
          event "保存": Value Change {
            w424 = "-"
            n157 = event-data() -> ()  [unwired: 2 out]
            n158 = Get Date/Time String(want seconds? (F)=TRUE) -> (date string=w402:string, time string=w425:string)  [unwired: 2 in]
            n159 = Search and Replace String(input string=w402, search string="/", replace string="-") -> (result string=w408:string)  [unwired: 5 in, 3 out]
            n160 = Search and Replace String(input string=w425, search string=":", replace string="-") -> (result string=w422:string)  [unwired: 5 in, 3 out]
            n161 = property on="保存_S" class="Bool (严格)"() -> ("Value"=w415:bool)  [unwired: 2 in, 2 out]
            n162 = Search and Replace String(input string=w408, search string="/", replace string="-") -> (result string=w403:string)  [unwired: 5 in, 3 out]
            n163 = Search and Replace String(input string=w422, search string=":", replace string="-") -> (result string=w423:string)  [unwired: 5 in, 3 out]
            n164 = Not(x=w415) -> (.not. x?=w410:bool)
            n165 = property on="保存_S" class="Bool (严格)"("Value"=w410) -> ()  [unwired: 2 in, 2 out]
            n166 = Concatenate Strings("D:\\PMSM\\", w403, w424, w423, w424, "电机数据存储", ".txt") -> (w412:string)
            n167 = Select(t=w412, s=w410, f="") -> (s? t:f=w417:string)
            n168 = String To Path(string=w417) -> (path=w401:path)
            n169 = local write "存储路径"(w401) -> ()
          }
          event "Close": Value Change {
            w437 = T10 1 items=["OK"=1, "ERROR1"=0, "ERROR2"=-1] ("y")
            n170 = event-data() -> ()  [unwired: 2 out]
            n171 = Unbundle By Name(w441) -> ("DevType"=w440:T5, "DevIndex"=w439:u32)
            n172 = call "VCI_CloseDevice.vi"("DevIndex"=w439, "DevType"=w440) -> ("Return Val"=w438:T10)  [unwired: 1 in, 8 out]
            n173 = Equal?(x=w438, y=w437) -> (x = y?=w435:bool)
            n174 = Not(x=w435) -> (.not. x?=w431:bool)
            n175 = Bundle By Name(cluster=cluster{"CANOpen":bool} {"CANOpen"=FALSE} ("事件数据"), "CANOpen"=w431) -> (w430:cluster{"CANOpen":bool})
            n176 = Bundle By Name(cluster=w436, "Open"=w431) -> (w434:cluster{"Open":bool, "SendCnt":u32})
            n177 = local write "Open"(w431) -> ()
            n178 = Generate User Event(user event=w433, event data cluster=w430) -> ()  [unwired: 1 in, 2 out]
          }
          event User Event {
            w451 = 0
            w450 = 0
            n179 = event-data() -> ("CANOpen"=w443:bool)  [unwired: 1 out]
            "Open" <- w443
            n180 = Not(x=w443) -> (.not. x?=w444:bool)
            n181 = Select(t=w450, s=w443, f=w451) -> (s? t:f=w452:i32)
            n182 = Select(t=w451, s=w443, f=w450) -> (s? t:f=w445:i32)
            n183 = property class="VI"("Front Panel.Closeable"=w444) -> ()  [unwired: 2 in, 2 out]
            n184 = property on="Close" class="Bool"("DisabledEnum"=w445) -> ()  [unwired: 2 in, 2 out]
            n185 = property on="ID" class="DigNum (严格)"("DisabledEnum"=w445) -> ()  [unwired: 2 in, 2 out]
            n186 = property on="Data" class="Str"("DisabledEnum"=w445) -> ()  [unwired: 2 in, 2 out]
            n187 = property on="Format" class="Ring (严格)"("DisabledEnum"=w445) -> ()  [unwired: 2 in, 2 out]
            n188 = property on="Type" class="Ring (严格)"("DisabledEnum"=w445) -> ()  [unwired: 2 in, 2 out]
            n189 = property on="Send" class="Bool"("DisabledEnum"=w445) -> ()  [unwired: 2 in, 2 out]
            n190 = Select(t=enum16{"Init", "Wait", "Run", "Exit"}."Run", s=w443, f=enum16{"Init", "Wait", "Run", "Exit"}."Wait") -> (s? t:f=w447:enum16{"Init", "Wait", "Run", "Exit"})
            n191 = property on="Fliter" class="Ring (严格)"("DisabledEnum"=w452) -> ()  [unwired: 2 in, 2 out]
            n192 = property on="DevType" class="Ring (严格)"("DisabledEnum"=w452) -> ()  [unwired: 2 in, 2 out]
            n193 = property on="Channel" class="Ring (严格)"("DisabledEnum"=w452) -> ()  [unwired: 2 in, 2 out]
            n194 = property on="AccCode" class="DigNum (严格)"("DisabledEnum"=w452) -> ()  [unwired: 2 in, 2 out]
            n195 = property on="AccMask" class="DigNum (严格)"("DisabledEnum"=w452) -> ()  [unwired: 2 in, 2 out]
            n196 = property on="InitFlag" class="Ring (严格)"("DisabledEnum"=w452) -> ()  [unwired: 2 in, 2 out]
            n197 = property on="Mode" class="Ring (严格)"("DisabledEnum"=w452) -> ()  [unwired: 2 in, 2 out]
            n198 = property on="kBaudRate" class="Ring (严格)"("DisabledEnum"=w452) -> ()  [unwired: 2 in, 2 out]
            n199 = property on="Open" class="Bool"("DisabledEnum"=w452) -> ()  [unwired: 2 in, 2 out]
          }
        }
      }
      frame "Exit" {
        n200 = Release Queue(queue=w463) -> ()  [unwired: 1 in, 4 out]
        n201 = Unregister For Events(event registration refnum=w462) -> (error out=w461:errorcluster)  [unwired: 1 in]
        n202 = Destroy User Event(user event=w460, error in=w461) -> ()  [unwired: 1 out]
        n203 = Unbundle By Name(w459) -> ("Open"=w458:bool)
        n204 = case shown="真" w458 {
          tunnel: w457 -> [_ w467]
          frame False {
          }
          frame True {
            n205 = Unbundle By Name(w467) -> ("DevType"=w466:T5, "DevIndex"=w465:u32)
            n206 = call "VCI_CloseDevice.vi"("DevIndex"=w465, "DevType"=w466) -> ()  [unwired: 1 in, 9 out]
          }
        }
        n207 = local write "RcvEnable"(FALSE ("RcvEnable")) -> ()
      }
    }
  }
  n208 = while "数据更新线程" {
    tunnel: w9 -> [w473]
    shift-right: [w468] -> _
    shift-left: u32 0 ("RecvCnt") -> [w469]
    stop <- w472 stop-if-true
    n209 = Dequeue Element(queue=w473) -> (element=w471:T7, timed out?=w470:bool, error out=w472:errorcluster)  [unwired: 2 in, 1 out]
    n210 = case shown="假" w470 {
      tunnel: w471 -> [w481 _]
      tunnel: w469 -> [w475 w679]
      tunnel: [w474 w679] -> w468
      frame False {
        n211 = Array To Cluster(array=w481) -> (cluster=w483:T12)
        n212 = Unbundle By Name(w483) -> ("[0]"=w482:T13)
        n213 = Increment(x=w475) -> (x+1=w474:u32)
        "sCnt" <- w474
        n214 = Unbundle By Name(w482) -> ("VCI_CAN_OBJ"=w480:T6)  [unwired: 3 out]
        n215 = Unbundle By Name(w480) -> ("ID"=w478:u32, "Data"=w479:u8[])  [unwired: 7 out]
        "CAN STD_ID" <- w478
        n216 = And(x=w478, y=u32 15) -> (x .and. y?=→"电机ID_R":u32)
        n217 = case shown="40" w478 {
          tunnel: w479 -> [_ w487]
          frame 0, Default {
          }
          frame 64 {
            n218 = local read "保存_S"() -> (w486:bool)
            n219 = local read "存储路径"() -> (w485:path)
            n220 = case shown="31" u32 49 {
              tunnel: w487 -> [_ w503 w539 w565 w581 w598 w612 w633 w650 w660 w670]
              tunnel: w486 -> [_ w498 _ _ _ _ _ _ _ _ _]
              tunnel: w485 -> [_ w493 _ _ _ _ _ _ _ _ _]
              frame 0, Default {
              }
              frame 49 {
                w505 = 8
                n221 = Array To Cluster(array=w503) -> (cluster=w510:T14)
                n222 = Unbundle By Name(w510) -> ("Data[1]"=w494:u8, "Data[2]"=w495:u8, "Data[3]"=w496:u8, "Data[4]"=w497:u8, "Data[5]"=w492:u8, "Data[6]"=w491:u8)  [unwired: 1 out]
                n223 = Join Numbers(hi=w492, lo=w491) -> ((hi.lo)=w490:u16)
                n224 = To Unsigned Word Integer(number=w494) -> (unsigned 16bit integer=w513:u16)
                n225 = To Unsigned Word Integer(number=w496) -> (unsigned 16bit integer=w509:u16)
                n226 = To Word Integer(number=w490) -> (16bit integer=w489:i16)
                n227 = Rotate(1:w513, 2:w505) -> (0:w512:u16)
                n228 = Rotate(1:w509, 2:w505) -> (0:w508:u16)
                n229 = Add(x=w512, y=w495) -> (x+y=w511:u16)
                n230 = Add(x=w508, y=w497) -> (x+y=w507:u16)
                n231 = Divide(x=w511, y=i16 1) -> (x/y=w501:dbl)
                "机械角度" <- w501
                n232 = Multiply(x=w507, y=0.0054931640625) -> (x*y=w500:dbl)
                "电气角度" <- w500
                n233 = Divide(x=w489, y=1.0) -> (x/y=w499:dbl)
                "转速" <- w499
                n234 = Build Array(w501, w500, w499) -> (w502:dbl[])
                n235 = case shown="真" w498 {
                  tunnel: w502 -> [_ w521]
                  tunnel: w493 -> [_ w514]
                  frame False {
                  }
                  frame True {
                    n236 = Open/Create/Replace File(file path (use dialog)=w514, operation (0:open)=T11."open or create") -> (refnum out=w524:refnum<file>)  [unwired: 4 in, 2 out]
                    n237 = for {
                      N: 3 -> [_]
                      shift-right: [w532] -> w520
                      shift-left: "" -> [w529]
                      tunnel: w521 -> [w528]
                      i -> [w527]
                      # "浮点文本存储"
                      # "2-14"
                      n238 = Index Array(array=w528, index=w527) -> (element=w526:dbl)
                      n239 = Number To Fractional String(number=w526) -> (F-format string=w531:string)  [unwired: 3 in]
                      n240 = Concatenate Strings(w529, w531, "\t") -> (w532:string)
                    }
                    n241 = Set File Position(refnum=w524, from (0:start)=u16 1) -> (refnum out=w523:refnum<file>)  [unwired: 2 in, 1 out]
                    n242 = Concatenate Strings(w520, "\r") -> (w518:string)
                    n243 = Write to Text File(file (use dialog)=w523, text=w518) -> (refnum out=w522:refnum<file>)  [unwired: 2 in, 2 out]
                    n244 = Close File(refnum=w522) -> ()  [unwired: 1 in, 2 out]
                  }
                }
              }
              frame 50 {
                w543 = i16 1024
                w544 = 8
                n245 = Array To Cluster(array=w539) -> (cluster=w551:T14)
                n246 = Unbundle By Name(w551) -> ("Data[1]"=w538:u8, "Data[2]"=w537:u8, "Data[3]"=w536:u8, "Data[4]"=w535:u8, "Data[5]"=w534:u8, "Data[6]"=w533:u8)  [unwired: 1 out]
                n247 = To Word Integer(number=w538) -> (16bit integer=w554:i16)
                n248 = To Word Integer(number=w534) -> (16bit integer=w547:i16)
                n249 = To Word Integer(number=w536) -> (16bit integer=w550:i16)
                n250 = Rotate(1:w554, 2:w544) -> (0:w553:i16)
                n251 = Rotate(1:w547, 2:w544) -> (0:w546:i16)
                n252 = Rotate(1:w550, 2:w544) -> (0:w549:i16)
                n253 = Add(x=w553, y=w537) -> (x+y=w552:i16)
                n254 = Add(x=w546, y=w533) -> (x+y=w545:i16)
                n255 = Add(x=w549, y=w535) -> (x+y=w548:i16)
                n256 = Divide(x=w552, y=w543) -> (x/y=→"A电流":dbl)
                n257 = Divide(x=w545, y=w543) -> (x/y=→"C电流":dbl)
                n258 = Divide(x=w548, y=w543) -> (x/y=→"B电流":dbl)
              }
              frame 51 {
                w567 = i16 256
                w566 = 8
                n259 = Array To Cluster(array=w565) -> (cluster=w574:T14)
                n260 = Unbundle By Name(w574) -> ("Data[1]"=w561:u8, "Data[2]"=w560:u8, "Data[3]"=w559:u8, "Data[4]"=w558:u8, "Data[5]"=w557:u8, "Data[6]"=w556:u8)  [unwired: 1 out]
                n261 = To Word Integer(number=w561) -> (16bit integer=w577:i16)
                n262 = To Word Integer(number=w559) -> (16bit integer=w573:i16)
                n263 = To Word Integer(number=w557) -> (16bit integer=w570:i16)
                n264 = Rotate(1:w577, 2:w566) -> (0:w576:i16)
                n265 = Rotate(1:w573, 2:w566) -> (0:w572:i16)
                n266 = Rotate(1:w570, 2:w566) -> (0:w569:i16)
                n267 = Add(x=w576, y=w560) -> (x+y=w575:i16)
                n268 = Add(x=w572, y=w558) -> (x+y=w571:i16)
                n269 = Add(x=w569, y=w556) -> (x+y=w568:i16)
                n270 = Divide(x=w575, y=i16 1024) -> (x/y=→"供电电压":dbl)
                n271 = Divide(x=w571, y=w567) -> (x/y=→"Ialfa":dbl)
                n272 = Divide(x=w568, y=w567) -> (x/y=→"Ibeta":dbl)
              }
              frame 52 {
                w580 = i16 256
                w586 = 8
                n273 = Array To Cluster(array=w581) -> (cluster=w590:T14)
                n274 = Unbundle By Name(w590) -> ("Data[1]"=w585:u8, "Data[2]"=w584:u8, "Data[3]"=w583:u8, "Data[4]"=w582:u8)  [unwired: 1 out]
                n275 = To Word Integer(number=w585) -> (16bit integer=w593:i16)
                n276 = To Word Integer(number=w583) -> (16bit integer=w589:i16)
                n277 = Rotate(1:w593, 2:w586) -> (0:w592:i16)
                n278 = Rotate(1:w589, 2:w586) -> (0:w588:i16)
                n279 = Add(x=w592, y=w584) -> (x+y=w591:i16)
                n280 = Add(x=w588, y=w582) -> (x+y=w587:i16)
                n281 = Divide(x=w591, y=w580) -> (x/y=→"Iqnow":dbl)
                n282 = Divide(x=w587, y=w580) -> (x/y=→"Idnow":dbl)
              }
              frame 53 {
                w602 = i16 1024
                w599 = 8
                n283 = Array To Cluster(array=w598) -> (cluster=w606:T14)
                n284 = Unbundle By Name(w606) -> ("Data[1]"=w597:u8, "Data[2]"=w596:u8, "Data[3]"=w595:u8, "Data[4]"=w594:u8)  [unwired: 1 out]
                n285 = To Word Integer(number=w597) -> (16bit integer=w609:i16)
                n286 = To Word Integer(number=w595) -> (16bit integer=w605:i16)
                n287 = Rotate(1:w609, 2:w599) -> (0:w608:i16)
                n288 = Rotate(1:w605, 2:w599) -> (0:w604:i16)
                n289 = Add(x=w608, y=w596) -> (x+y=w607:i16)
                n290 = Add(x=w604, y=w594) -> (x+y=w603:i16)
                n291 = Divide(x=w607, y=w602) -> (x/y=→"Uq":dbl)
                n292 = Divide(x=w603, y=w602) -> (x/y=→"Ud":dbl)
              }
              frame 54 {
                w618 = i16 1024
                w617 = 8
                n293 = Array To Cluster(array=w612) -> (cluster=w622:T14)
                n294 = Unbundle By Name(w622) -> ("Data[1]"=w616:u8, "Data[2]"=w615:u8, "Data[3]"=w614:u8, "Data[4]"=w613:u8)  [unwired: 1 out]
                n295 = To Word Integer(number=w616) -> (16bit integer=w625:i16)
                n296 = To Word Integer(number=w614) -> (16bit integer=w621:i16)
                n297 = Rotate(1:w625, 2:w617) -> (0:w624:i16)
                n298 = Rotate(1:w621, 2:w617) -> (0:w620:i16)
                n299 = Add(x=w624, y=w615) -> (x+y=w623:i16)
                n300 = Add(x=w620, y=w613) -> (x+y=w619:i16)
                n301 = Divide(x=w623, y=w618) -> (x/y=→"Ualfa":dbl)
                n302 = Divide(x=w619, y=w618) -> (x/y=→"Ubate":dbl)
              }
              frame 55 {
                w638 = u16 0
                w637 = 8
                n303 = Array To Cluster(array=w633) -> (cluster=w645:T14)
                n304 = Unbundle By Name(w645) -> ("Data[1]"=w626:u8, "Data[2]"=w627:u8, "Data[3]"=w628:u8, "Data[4]"=w629:u8, "Data[5]"=w630:u8, "Data[6]"=w631:u8, "Data[7]"=→"sector":u8)  [unwired: 1 out]
                n305 = To Word Integer(number=w626) -> (16bit integer=w648:i16)
                n306 = To Word Integer(number=w628) -> (16bit integer=w644:i16)
                n307 = To Word Integer(number=w630) -> (16bit integer=w641:i16)
                n308 = Rotate(1:w648, 2:w637) -> (0:w647:i16)
                n309 = Rotate(1:w644, 2:w637) -> (0:w643:i16)
                n310 = Rotate(1:w641, 2:w637) -> (0:w640:i16)
                n311 = Add(x=w647, y=w627) -> (x+y=w646:i16)
                n312 = Add(x=w643, y=w629) -> (x+y=w642:i16)
                n313 = Add(x=w640, y=w631) -> (x+y=w639:i16)
                n314 = Subtract ("减")(x=w646, y=w638) -> (x-y=→"PWM1":u16)
                n315 = Subtract ("减")(x=w642, y=w638) -> (x-y=→"PWM2":u16)
                n316 = Subtract ("减")(x=w639, y=w638) -> (x-y=→"PWM3":u16)
              }
              frame 64 {
                n317 = Array To Cluster(array=w650) -> (cluster=w655:T14)
                n318 = Unbundle By Name(w655) -> ("Data[1]"=w651:u8, "Data[2]"=w652:u8)  [unwired: 1 out]
                n319 = To Unsigned Word Integer(number=w651) -> (unsigned 16bit integer=w658:u16)
                n320 = Rotate(1:w658, 2:8) -> (0:w657:u16)
                n321 = Add ("加")(x=w657, y=w652) -> (x+y=w656:u16)
                n322 = Divide(x=w656, y=u16 256) -> (x/y=→"设定位置_回":dbl)
              }
              frame 65 {
                n323 = Array To Cluster(array=w660) -> (cluster=w665:T14)
                n324 = Unbundle By Name(w665) -> ("Data[1]"=w661:u8, "Data[2]"=w662:u8)  [unwired: 1 out]
                n325 = To Unsigned Word Integer(number=w661) -> (unsigned 16bit integer=w668:u16)
                n326 = Rotate(1:w668, 2:8) -> (0:w667:u16)
                n327 = Add ("加")(x=w667, y=w662) -> (x+y=w666:u16)
                n328 = Divide(x=w666, y=u16 1) -> (x/y=→"设定速度_回":dbl)
              }
              frame 66 {
                n329 = Array To Cluster(array=w670) -> (cluster=w675:T14)
                n330 = Unbundle By Name(w675) -> ("Data[1]"=w671:u8, "Data[2]"=w672:u8)  [unwired: 1 out]
                n331 = To Word Integer(number=w671) -> (16bit integer=w678:i16)
                n332 = Rotate(1:w678, 2:8) -> (0:w677:i16)
                n333 = Add ("加")(x=w677, y=w672) -> (x+y=w676:i16)
                n334 = Divide(x=w676, y=u16 256) -> (x/y=→"设定电流_回":dbl)
              }
            }
          }
        }
      }
      frame True {
      }
    }
  }
  n335 = while "接收线程" {
    tunnel: w9 -> [w682]
    shift-right: [w680] -> _
    shift-left: u32 0 ("RecvCnt") -> [w681]
    stop <- "RcvEnable" continue-if-true
    n336 = local read "Open"() -> (w683:bool)
    n337 = case shown="真" w683 {
      tunnel: w682 -> [_ w690]
      tunnel: w681 -> [w685 w689]
      tunnel: [w685 w688] -> w680
      frame False {
        # "CAN未打开，延时50ms"
        n338 = Wait (ms)(milliseconds to wait=u32 50 ("等待时间（毫秒）")) -> ()  [unwired: 1 out]
      }
      frame True {
        n339 = local read "DevType"() -> (w694:T5)
        n340 = local read "Channel"() -> (w687:T4)
        n341 = call "VCI_Receive.vi"("CANIndex"=w687, "DevIndex"=u32 0, "DevType"=w694) -> ("Recieve"=w691:T6[])  [unwired: 3 in, 5 out]
        n342 = Empty Array?(array=w691) -> (empty?=w692:bool)
        n343 = case shown="假" w692 {
          tunnel: w690 -> [w703 _]
          tunnel: w691 -> [w699 _]
          tunnel: [w700 _] -> _
          tunnel: w689 -> [w697 w704]
          tunnel: [w696 w704] -> w688
          tunnel: w687 -> [w695 _]
          frame False {
            n344 = Array Size(array=w699) -> (size(s)=w698:i32)
            n345 = call "Demo_MakeDispBuff.vi"("Channel"=w695, "Type"=enum16{"接收", "发送"}."接收", "OBJs"=w699) -> ("Buffer"=w701:T7)
            n346 = Add(x=w698, y=w697) -> (x+y=w696:u32)
            "RecvCnt" <- w696
            n347 = Enqueue Element(queue=w703, element=w701) -> (error out=w700:errorcluster)  [unwired: 1 in, 3 out]
          }
          frame True {
          }
        }
      }
    }
  }
  n348 = control-ref of="本应用程序"() -> (w6:refnum<vi>)
  n349 = invoke class="VI" method="FP.Close"(error in=w4) -> (error out=w3:errorcluster)  [unwired: 2 in, 2 out]
  n350 = property class="App"(reference=w6) -> ("App.Kind"=w5:T15)  [unwired: 1 in, 2 out]
  n351 = case shown="\"Development System\"" w5 {
    tunnel: w3 -> [_ _]
    frame "invalid app kind", Default {
      n352 = Quit LabVIEW() -> ()  [unwired: 1 out]
    }
    frame "Development System" {
    }
  }
